vi "CubeSwitcher.vi"(8 "error in (no error)":errorcluster, 10 "Ring":u16(ring) items=["1", "2", "3"]) -> (0 "error out":errorcluster)   [LabVIEW 2015]
panel:
  out "return count":u32
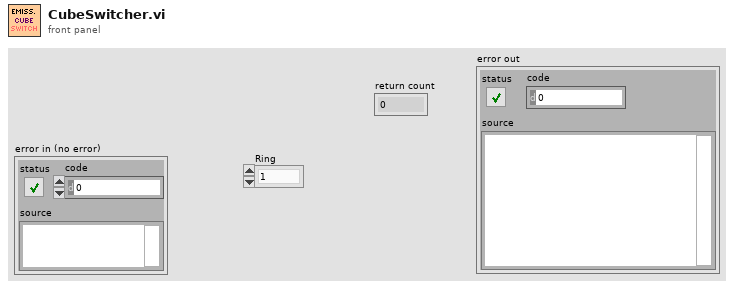
[diagram p1: front panel]
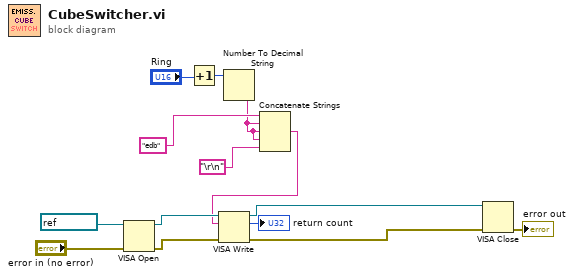
[diagram p0: block diagram]
diagram:
  n1 = VISA Open(error in (no error)="error in (no error)", VISA resource name=refnum<visa-resource-name> "COM1") -> (VISA resource name=w11:refnum<visa-resource-name>, error out=w12:errorcluster)  [unwired: 3 in]
  n2 = Increment(x="Ring") -> (x+1=w3:u16)
  n3 = Number To Decimal String(number=w3) -> (decimal integer string=w2:string)  [unwired: 1 in]
  n4 = Concatenate Strings("edb", w2, w2, w2, "\r\n") -> (w9:string)
  n5 = VISA Write(VISA resource name=w11, write buffer=w9, error in (no error)=w12) -> (VISA resource name out=w7:refnum<visa-resource-name>, return count=→"return count":u32, error out=w6:errorcluster)
  n6 = VISA Close(VISA resource name=w7, error in (no error)=w6) -> (error out=→"error out":errorcluster)
